vi "Parse geAll.vi"(8 "error in (no error)":errorcluster, 10 "getAll":variant) -> (0 "error out":errorcluster, 2 "getAll cluster":T7)   [LabVIEW 2016, in "SR7270 UI.lvclass"]
uses:
  SR7270 UI.lvclass
  Instrument.SR7270/Driver/Typedefs/VMODE--enum.ctl
  Instrument.SR7270/Driver/Typedefs/IMODE--enum.ctl
  Instrument.SR7270/Driver/Typedefs/FLOAT--enum.ctl
  Instrument.SR7270/Driver/Typedefs/FET--enum.ctl
  Instrument.SR7270/Driver/Typedefs/LF--enum.ctl
  Instrument.SR7270/Driver/Typedefs/SEN-IMODE0--enum.ctl
  Instrument.SR7270/Typedefs/getAll.ctl
  Instrument.SR7270/Driver/SR7270 Drivers.lvlib
  Instrument.SR7270/Instrument.SR7270.lvclass
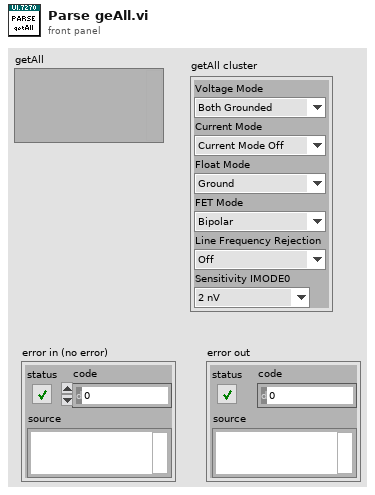
[diagram p1: front panel]
types:
  T1 = typedef "SR7270 Drivers.lvlib/VMODE--enum.ctl" = enum16{"Both Grounded", "A input only", "-B input only", "A-B differential"}
  T2 = typedef "SR7270 Drivers.lvlib/IMODE--enum.ctl" = enum16{"Current Mode Off", "High bandwidth current mode", "Low noise current mode"}
  T3 = typedef "SR7270 Drivers.lvlib/FLOAT--enum.ctl" = enum16{"Ground", "Float"}
  T4 = typedef "SR7270 Drivers.lvlib/FET--enum.ctl" = enum16{"Bipolar", "FET"}
  T5 = typedef "SR7270 Drivers.lvlib/LF--enum.ctl" = enum16{"Off", "60 Hz", "120 Hz", "60 & 120 Hz"}
  T6 = typedef "SR7270 Drivers.lvlib/SEN-IMODE0--enum.ctl" = enum16{"2 nV", "5 nV", "10 nV", "20 nV", "50 nV", "100 nV", "200 nV", "500 nV", "1 µV", "2 µV", "5 µV", "10 µV", "20 µV", "50 µV", "100 µV", "200 µV", "500 µV", "1 mV", "2 mV", "5 mV", "10 mV", "20 mV", "50 mV", "100 mV", "200 mV", "500 mV", "1 V"}
  T7 = cluster{"Voltage Mode":T1, "Current Mode":T2, "Float Mode":T3, "FET Mode":T4, "Line Frequency Rejection":T5, "Sensitivity IMODE0":T6}
  T8 = typedef "Instrument.SR7270.lvclass/getAll.ctl" = cluster{"X (V or A)":dbl, "Y (V or A)":dbl, "Mag (V or A)":dbl, "Phase (°)":dbl, "Oscillator Amplitude (V)":dbl, "Oscillator frequency (Hz)":dbl, "REF time constant (s)":dbl, "REF harmonic":u16, "REF phase (°)":dbl, "REF frequency (Hz)":dbl, "AC Gain":string, "Current Mode":string, "AC-DC Coupling":string, "FET":string, "Float":string, "Line Filter":string, "Voltage Mode":string, "Sensitivity (V or A)":dbl}
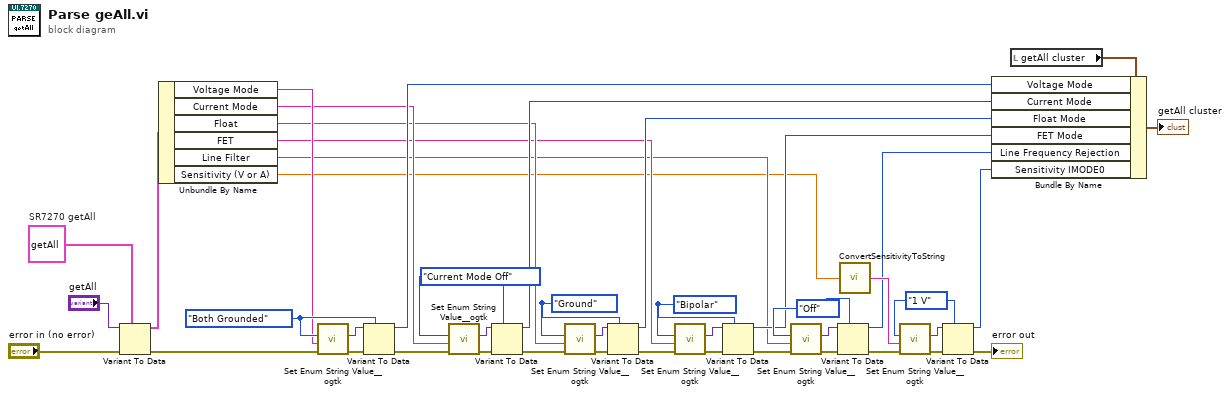
[diagram p0: block diagram]
diagram:
  w34 = LF--enum."Off" ("Line Frequency Rejection")
  w16 = FET--enum."Bipolar" ("FET Mode")
  w15 = FLOAT--enum."Ground" ("Float Mode")
  w14 = IMODE--enum."Current Mode Off" ("Current Mode")
  w13 = VMODE--enum."Both Grounded" ("Voltage Mode")
  w39 = T8 {"X (V or A)"=0.0, "Y (V or A)"=0.0, "Mag (V or A)"=0.0, "Phase (°)"=0.0, "Oscillator Amplitude (V)"=0.0, "Oscillator frequency (Hz)"=0.0, "REF time constant (s)"=0.0, "REF harmonic"=0, "REF phase (°)"=0.0, "REF frequency (Hz)"=0.0, "AC Gain"="", "Current Mode"="", "AC-DC Coupling"="", "FET"="", "Float"="", "Line Filter"="", "Voltage Mode"="", "Sensitivity (V or A)"=0.0}  # SR7270 getAll
  w42 = SEN-IMODE0--enum."1 V" ("Sensitivity IMODE0")
  n1 = Variant To Data(error in="error in (no error)", type=w39, Variant="getAll") -> (data=w44:T8, error out=w23:errorcluster)
  n2 = Unbundle By Name(w44) -> ("Voltage Mode"=w6:string, "Current Mode"=w5:string, "Float"=w4:string, "FET"=w3:string, "Line Filter"=w2:string, "Sensitivity (V or A)"=w1:dbl)
  n3 = call <userlib>:"Set Enum String Value__ogtk.vi"("error in (no error)"=w23, "String Value"=w6, "Default Enum Value"=w13) -> ("error out"=w31:errorcluster, "Enum"=w32:variant)  [unwired: 7 in]
  n4 = Variant To Data(error in=w31, type=w13, Variant=w32) -> (data=w12:T1, error out=w22:errorcluster)
  n5 = call <userlib>:"Set Enum String Value__ogtk.vi"("error in (no error)"=w22, "String Value"=w5, "Default Enum Value"=w14) -> ("error out"=w29:errorcluster, "Enum"=w30:variant)  [unwired: 7 in]
  n6 = Variant To Data(error in=w29, type=w14, Variant=w30) -> (data=w11:T2, error out=w21:errorcluster)
  n7 = call <userlib>:"Set Enum String Value__ogtk.vi"("error in (no error)"=w21, "String Value"=w4, "Default Enum Value"=w15) -> ("error out"=w27:errorcluster, "Enum"=w28:variant)  [unwired: 7 in]
  n8 = Variant To Data(error in=w27, type=w15, Variant=w28) -> (data=w10:T3, error out=w20:errorcluster)
  n9 = call <userlib>:"Set Enum String Value__ogtk.vi"("error in (no error)"=w20, "String Value"=w3, "Default Enum Value"=w16) -> ("error out"=w25:errorcluster, "Enum"=w26:variant)  [unwired: 7 in]
  n10 = Variant To Data(error in=w25, type=w16, Variant=w26) -> (data=w9:T4, error out=w19:errorcluster)
  n11 = call <userlib>:"Set Enum String Value__ogtk.vi"("error in (no error)"=w19, "String Value"=w2, "Default Enum Value"=w34) -> ("error out"=w24:errorcluster, "Enum"=w33:variant)  [unwired: 7 in]
  n12 = Variant To Data(error in=w24, type=w34, Variant=w33) -> (data=w8:T5, error out=w18:errorcluster)
  n13 = call "ConvertSensitivityToString.vi"("Sensitivity"=w1) -> ("Sensitivity String"=w43:string)
  n14 = call <userlib>:"Set Enum String Value__ogtk.vi"("error in (no error)"=w18, "String Value"=w43, "Default Enum Value"=w42) -> ("error out"=w40:errorcluster, "Enum"=w41:variant)  [unwired: 7 in]
  n15 = Variant To Data(error in=w40, type=w42, Variant=w41) -> (data=w7:T6, error out=→"error out":errorcluster)
  n16 = local read "getAll cluster"() -> (w36:T7)
  n17 = Bundle By Name(cluster=w36, "Voltage Mode"=w12, "Current Mode"=w11, "Float Mode"=w10, "FET Mode"=w9, "Line Frequency Rejection"=w8, "Sensitivity IMODE0"=w7) -> (→"getAll cluster":T7)
